vi "svfa_Scaled Time Domain Window (1xM) (Dual).vi"(0 "stimulus signals X [EUx]":waveform(dbl)[](array[waveform]), 5 "response signal Y [EUy]":waveform(dbl), 7 "window":T1 items=["None"=0, "Hanning"=1, "Hamming"=2, "Blackman-Harris"=3, "Exact Blackman"=4, "Blackman"=5, "Flat Top"=6, "4 Term B-Harris "=7, "7 Term B-Harris"=8, "Low Sidelobe"=9, "Force - Exponential"=10, "Blackman Nuttall"=11, "Triangle"=30, "Bartlett-Hanning"=31, "Bohman"=32, "Parzen"=33, "Welch"=34, "Kaiser"=60, "Dolph-Chebyshev"=61, "Gaussian"=62], 9 "force and exponential window settings":cluster{"force [%]":dbl, "exponential [%]":dbl}={"force [%]"=50.0, "exponential [%]"=10.0} {"exponential [%]" min=0.0 max=100.0 format="%.2f"; "force [%]" min=0.0 max=100.0 format="%.2f"}, 11 "error in (no error)":errorcluster) -> (4 "stimulus signals X [EUx]":waveform(dbl)[](array[waveform]), 6 "response signal Y [EUy]":waveform(dbl), 8 "window":u16(ring) items=["None "=0, "Hanning"=1, "Hamming"=2, "Blackman-Harris"=3, "Exact Blackman"=4, "Blackman"=5, "Flat Top"=6, "4 Term B-Harris "=7, "7 Term B-Harris"=8, "Low Sidelobe"=9, "Force - Exponential"=10, "Gaussian"=62], 10 "window size":i32, 15 "error out":errorcluster)   [LabVIEW 2017]
doc: "Applies the selected window to the time-domain signal. The VI scales the result so that when the power or amplitude spectrum of the windowed waveform is computed, all windows provide the same level within the accuracy constraints of the window."
uses:
  <vilib>/addons/_NISVFA/_Shared subVIs/Controls/svc_Window [Dual FFT].ctl
  <vilib>/addons/_NISVFA/_Shared subVIs/Windowing/svfa_Scaled Time Domain Window (Array).vi
  <vilib>/Analysis/4window.llb/Force Window.vi
  <vilib>/Analysis/4window.llb/Force Window (DBL).vi
  <vilib>/Analysis/4window.llb/Exponential Window.vi
  <vilib>/Analysis/4window.llb/Exponential Window (DBL).vi
  <vilib>/Utility/error.llb/Error Cluster From Error Code.vi
  <vilib>/Analysis/0measdsp.llb/Scaled Time Domain Window.vi
  <vilib>/Analysis/0measdsp.llb/Scaled Time Domain Window (DBL).vi
  <vilib>/addons/_NISVFA/_Spectrum Processing/subVIs/svfa_Spectrum Info Window to windowTd Type Def.vi
  <vilib>/addons/_NISVFA/_Shared subVIs/Common/svc_Window Parameters.vi
  <vilib>/addons/_NISVFA/_Shared subVIs/Common/svc_Get Window Info.vi
panel:
  # "Scaled Time Domain Window"
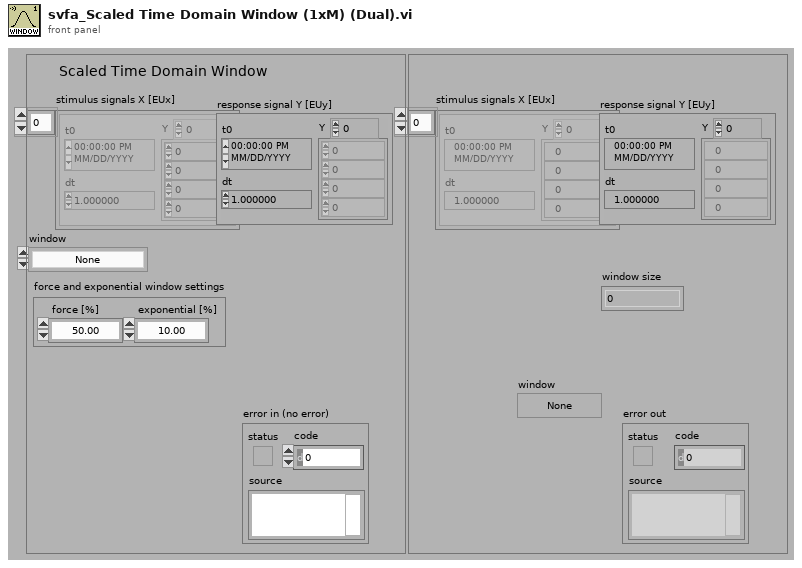
[diagram p1: front panel]
types:
  T1 = typedef "svc_Window [Dual FFT].ctl" = u32
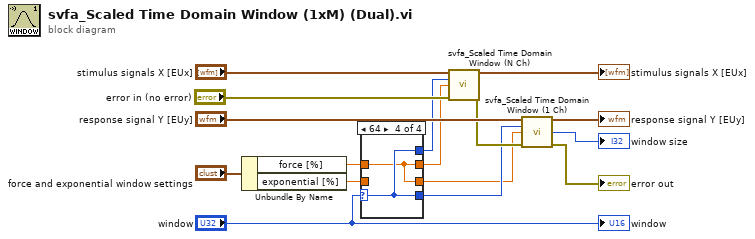
[diagram p0: block diagram]
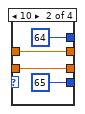
[diagram p3: hidden frame]
diagram:
  n1 = Unbundle By Name("force and exponential window settings") -> ("force [%]"=w3:dbl, "exponential [%]"=w1:dbl)
  n2 = case shown="64" "window" {
    selector: "window" -> [w19 _ w25 w27]
    tunnel: [w19 u16 64 ("window") w25 w27] -> w6
    tunnel: [w19 u16 65 ("window") w25 w27] -> w7
    tunnel: [w18 w21 w24 w26] -> w4
    tunnel: w3 -> [w18 w21 _ w26]
    tunnel: [w17 w20 w24 w26] -> w2
    tunnel: w1 -> [w17 w20 w24 _]
    frame 0, Default {
    }
    frame 10 {
    }
    frame 65 {
    }
    frame 64 {
    }
  }
  n3 = call <vilib>:"svfa_Scaled Time Domain Window (N Ch).vi"("Scaled signal(s)"="stimulus signals X [EUx]", "window"=w6, "window parameter"=w4, "error in (no error)"="error in (no error)") -> ("Windowed Waveform(s)"=→"stimulus signals X [EUx]":waveform(dbl)[], "error out"=w9:errorcluster)  [unwired: 7 in, 3 out]
  n4 = call <vilib>:"svfa_Scaled Time Domain Window (1 Ch).vi"("Signal in [X]"="response signal Y [EUy]", "window"=w7, "window parameter"=w2, "error in"=w9) -> ("Windowed Waveform"=→"response signal Y [EUy]":waveform(dbl), "window length"=→"window size":i32, "error out"=→"error out":errorcluster)  [unwired: 6 in, 3 out]
  "window" <- "window"
